vi "setUp.vi"(8 "error in (no error)":errorcluster, 11 "reference in":refnum<class "SMO_TestSuite.lvclass">) -> (0 "error out":errorcluster, 3 "reference out":refnum<class "SMO_TestSuite.lvclass">)   [LabVIEW 2013, in "SMO_TestSuite.lvclass"]
doc: "setUp runs prior to the test method during test execution. Use this method to initialize any object data required by your tests."
uses:
  SMO_TestSuite.lvclass
  SMO_TestSuite.lvclass/SMO_TestSuite.ctl
  <vilib>/addons/_JKI Toolkits/VI Tester/TestSuite.llb/TestSuite.lvclass
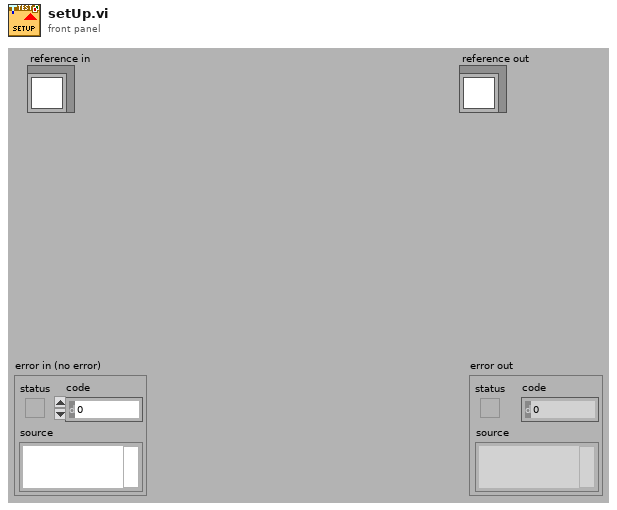
[diagram p1: front panel]
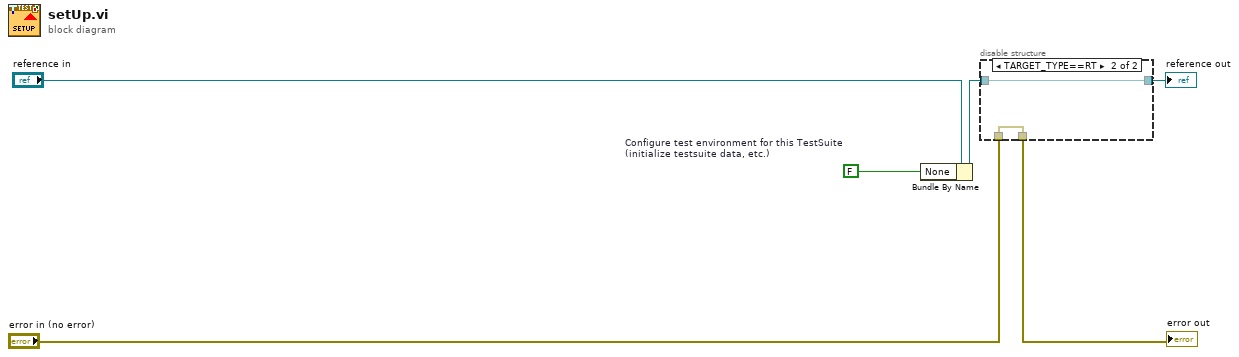
[diagram p0: block diagram]
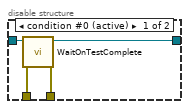
[diagram p2: hidden frame]
diagram:
  w5 = FALSE  # Configure test environment for this TestSuite  (initialize testsuite data, etc.)
  n1 = Bundle By Name(cluster="reference in", "None"=w5) -> (w4:refnum<class "SMO_TestSuite.lvclass">)
  n2 = disable-structure shown="TARGET_TYPE==RT" {
    disable-tunnel: w4 -> [w10 w11]
    disable-tunnel: [w9 w11] -> w3
    disable-tunnel: "error in (no error)" -> [w8 w12]
    disable-tunnel: [w7 w12] -> w1
    frame condition #0 (active) {
      n3 = call <vilib>:"WaitOnTestComplete.vi"("error in (no error)"=w8, "TestSuite in"=w10) -> ("error out"=w7:errorcluster, "TestSuite out"=w9:refnum<class "SMO_TestSuite.lvclass">)  [unwired: 8 in]
    }
    frame condition #1 {
    }
  }
  "error out" <- w1
  "reference out" <- w3
